vi "initialize_instruments (SubVI).vi"(1 "Sample rate":dbl=1000.0 format="%0.2f", 5 "Electrode outupt channels":tag="Dev4/ao0", 7 "make volt file":bool, 9 "volt file path":path, 12 "Step Picomotors?":bool) -> (4 "analog_out_config":T1, 6 "Volt vs pos array":cluster{dbl, dbl}[](array[cluster]), 15 "Picomotor Instr":T2)   [LabVIEW 2022 SP3]
uses:
  C:/Program Files (x86)/New Focus/New Focus Picomotor Application/Samples/LabVIEW/Model 8742/LabVIEW 2009/CmdLib.dll
  Program Files (x86)/New Focus/New Focus Picomotor Application/Samples/LabVIEW/Model 8742/LabVIEW 2009/CmdLib.dll
  <vilib>/DAQmx/create/channels.llb/DAQmx Create Channel (AO-Voltage-Basic).vi
  <vilib>/Utility/file.llb/Read From Spreadsheet File (DBL).vi
  <vilib>/DAQmx/configure/timing.llb/DAQmx Timing (Sample Clock).vi
  <resource>/objmgr/daqmx.rc
panel:
  out "SampClk.Rate":dbl
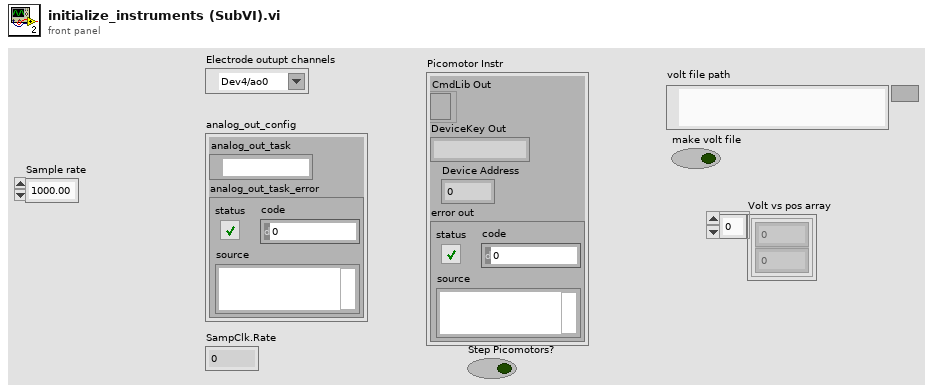
[diagram p1: front panel]
types:
  T1 = cluster{"analog_out_task":refnum<k21>, "analog_out_task_error":errorcluster}
  T2 = cluster{"CmdLib Out":refnum<k24>, "DeviceKey Out":string, "Device Address":i32, "error out":errorcluster}
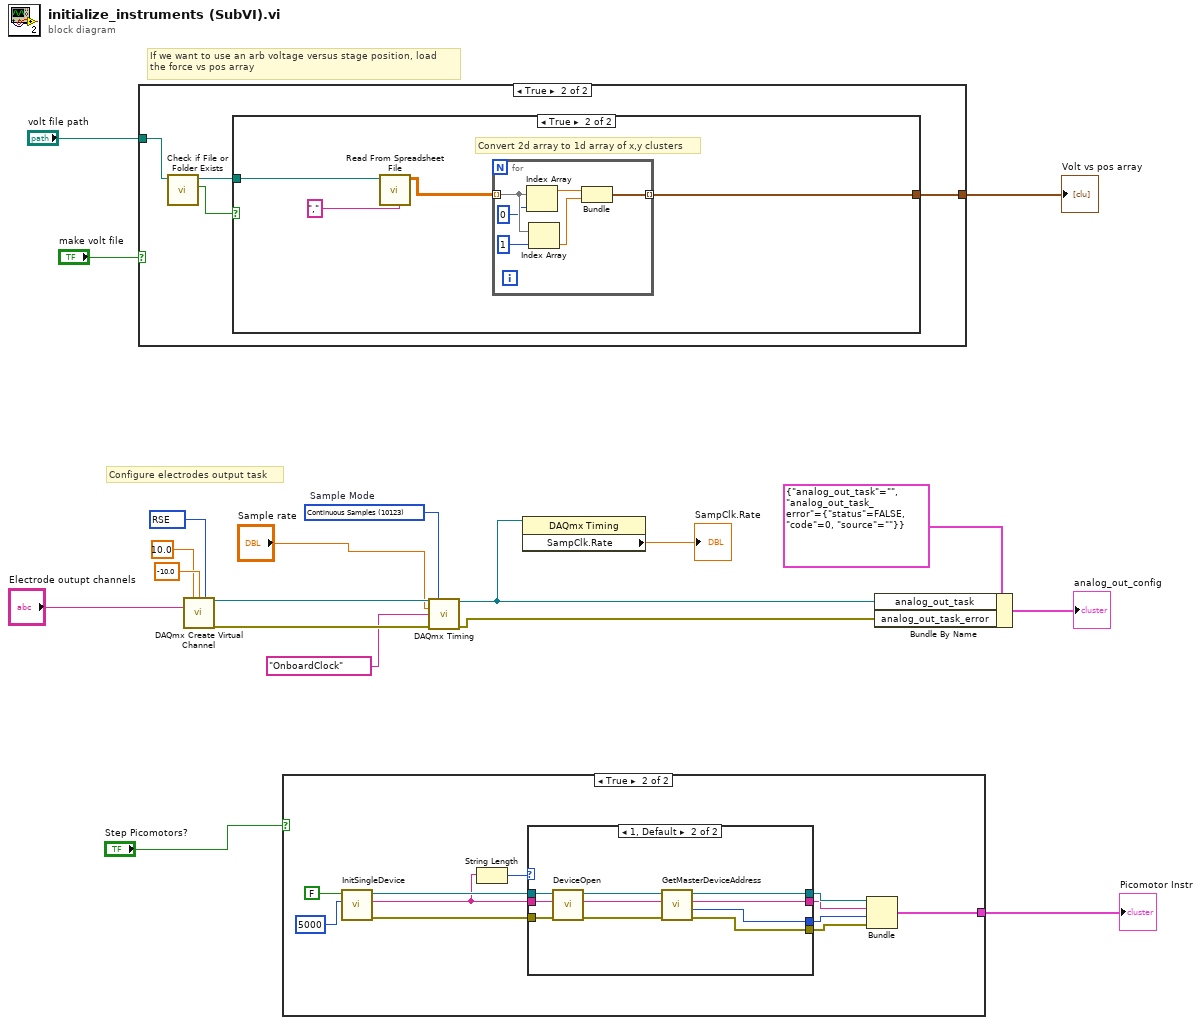
[diagram p0: block diagram]
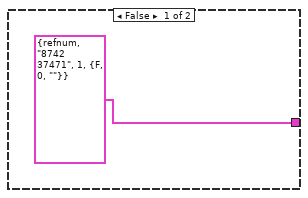
[diagram p2: hidden frame]
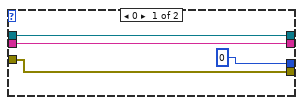
[diagram p3: hidden frame]
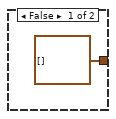
[diagram p4: hidden frame]
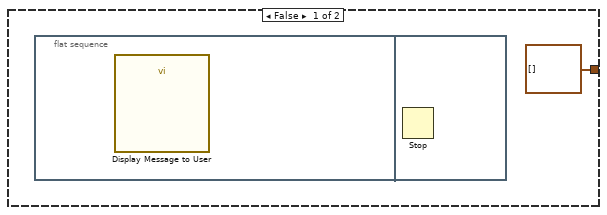
[diagram p5: hidden frame]
diagram:
  w14 = 10083 items=["Default"=-1, "RSE"=10083, "Differential"=10106, "Pseudodifferential"=12529] ("output terminal configuration")
  w19 = 10123 items=["Finite Samples"=10178, "Continuous Samples"=10123, "Hardware Timed Single Point"=12522]  # Sample Mode
  # "If we want to use an arb voltage versus stage position, load\nthe force vs pos array"
  # "Configure electrodes output task"
  n1 = case shown="True" "make volt file" {
    tunnel: "volt file path" -> [_ w23]
    tunnel: [cluster{dbl, dbl}[] [] w21] -> w8
    frame False {
    }
    frame True {
      n2 = call <vilib>:"Check if File or Folder Exists.vi"("path"=w23) -> ("file or folder exists?"=w24:bool, "dup path"=w22:path)  [unwired: 8 in, 1 out]
      n3 = case shown="True" w24 {
        tunnel: w22 -> [_ w28]
        tunnel: [cluster{dbl, dbl}[] [] w26] -> w21
        frame False {
          n4 = flat-sequence {
            frame #0 {
              n5 = call "Display Message to User"() -> ()  [unwired: 10 in, 2 out]
            }
            frame #1 {
              n6 = Stop() -> ()  [unwired: 1 in]
            }
          }
        }
        frame True {
          # "Convert 2d array to 1d array of x,y clusters"
          n7 = call-poly <vilib>:"Read From Spreadsheet File.vi"("delimiter (\\t)"="," ("delimiter (\\t)"), "file path (dialog if empty)"=w28) -> ("all rows"=w27:dbl[][])  [unwired: 5 in, 4 out]
          n8 = for {
            tunnel: w27 -> [w35] mode=indexing
            tunnel: [w30] -> w26 mode=indexing
            n9 = Index Array(array=w35, index=0) -> (element=w32:dbl)
            n10 = Index Array(array=w35, index=1) -> (element=w31:dbl)
            n11 = Bundle(w32, w31) -> (w30:cluster{dbl, dbl})  [unwired: 1 in]
          }
        }
      }
    }
  }
  "Volt vs pos array" <- w8
  n12 = call-poly <vilib>:"DAQmx Create Virtual Channel.vi"("maximum value"=10.0, "minimum value"=-10.0, "output terminal configuration"=w14, "physical channels"="Electrode outupt channels") -> ("task out"=w17:refnum<k21>, "error out"=w18:errorcluster)  [unwired: 10 in]
  n13 = case shown="True" "Step Picomotors?" {
    tunnel: [T2 {"CmdLib Out"=refnum, "DeviceKey Out"="8742 37471", "Device Address"=1, "error out"={"status"=FALSE, "code"=0, "source"=""}} ("Picomotor Instr 2") w37] -> w6
    frame False {
    }
    frame True {
      n14 = call <instrlib>:"InitSingleDevice.vi"("msecDelayForDiscovery"=5000, "logging"=FALSE) -> ("error out"=w42:errorcluster, "DeviceKey Out"=w43:string, "CmdLib Out"=w44:refnum<k24>)  [unwired: 3 in]
      n15 = String Length(string=w43) -> (length=w45:i32)
      n16 = case shown="1, Default" w45 {
        tunnel: w44 -> [w51 w58]
        tunnel: w43 -> [w50 w57]
        tunnel: w42 -> [w49 w56]
        tunnel: [w51 w55] -> w41
        tunnel: [w50 w54] -> w40
        tunnel: [0 ("msecDelayForDiscovery") w53] -> w39
        tunnel: [w49 w52] -> w38
        frame 0 {
        }
        frame 1, Default {
          n17 = call <instrlib>:"DeviceOpen.vi"("error in (no error)"=w56, "DeviceKey In"=w57, "CmdLib In"=w58) -> ("error out"=w61:errorcluster, "DeviceKey Out"=w60:string, "CmdLib Out"=w59:refnum<k24>)  [unwired: 2 in]
          n18 = call <instrlib>:"GetMasterDeviceAddress.vi"("error in (no error)"=w61, "DeviceKey In"=w60, "CmdLib In"=w59) -> ("error out"=w52:errorcluster, "Device Address"=w53:i32, "DeviceKey Out"=w54:string, "CmdLib Out"=w55:refnum<k24>)  [unwired: 1 in]
        }
      }
      n19 = Bundle("CmdLib Out"=w41, "DeviceKey Out"=w40, "Device Address"=w39, "error out"=w38) -> (w37:T2)  [unwired: 1 in]
    }
  }
  "Picomotor Instr" <- w6
  n20 = call-poly <vilib>:"DAQmx Timing.vi"("task/channels in"=w17, "sample mode"=w19, "rate"="Sample rate", "source"=tag "OnboardClock" ("Sample Clock Source"), "error in"=w18) -> ("task out"=w4:refnum<k21>, "error out"=w2:errorcluster)  [unwired: 9 in]
  n21 = property class="DAQmx Timing"(reference=w4) -> ("SampClk.Rate"=→"SampClk.Rate":dbl)  [unwired: 1 in, 2 out]
  n22 = Bundle By Name(cluster=T1 {"analog_out_task"="", "analog_out_task_error"={"status"=FALSE, "code"=0, "source"=""}} ("input cluster"), "analog_out_task"=w4, "analog_out_task_error"=w2) -> (→"analog_out_config":T1)
